vi "Func-엑셀 데이터를 그래프로 출력.vi"() -> ()   [LabVIEW 2015] (continued)
-12.31\n-18.3\t-18.31\t-12.305\n-18.3\t-18.31\t-12.3\n-18.3\t-18.31\t-12.299\n-18.3\t-18.31\t-12.293\n-18.3\t-18.31\t-12.295\n-18.3\t-18.31\t-12.293\n-18.3\t-18.31\t-12.286\n-18.3\t-18.31\t-12.284\n-18.3\t-18.31\t-12.277\n-18.3\t-18.31\t-12.27\n-18.3\t-18.31\t-12.265\n-18.3\t-18.31\t-12.259\n-18.3\t-18.31\t-12.253\n-18.3\t-18.31\t-12.251\n-18.3\t-18.31\t-12.25\n-18.3\t-18.31\t-12.245\n-18.3\t-18.31\t-12.239\n-18.3\t-18.31\t-12.232\n-18.3\t-18.31\t-12.23\n-18.3\t-18.31\t-12.226\n-18.3\t-18.31\t-12.221\n-18.3\t-18.31\t-12.22\n-18.3\t-18.31\t-12.216\n-18.3\t-18.31\t-12.214\n-18.3\t-18.31\t-12.209\n-18.3\t-18.31\t-12.205\n-18.3\t-18.31\t-12.202\n-18.3\t-18.31\t-12.199\n-18.3\t-18.31\t-12.195\n-18.3\t-18.31\t-12.192\n-18.3\t-18.31\t-12.186\n-18.3\t-18.31\t-12.184\n-18.3\t-18.31\t-12.179\n-18.3\t-18.31\t-12.169\n-18.3\t-18.31\t-12.166\n-18.3\t-18.31\t-12.161\n-18.3\t-18.31\t-12.157\n-18.3\t-18.31\t-12.152\n-18.3\t-18.31\t-12.15\n-18.3\t-18.31\t-12.146\n-18.3\t-18.31\t-12.143\n-18.3\t-18.31\t-12.142\n-18.3\t-18.31\t-12.137\n-18.3\t-18.31\t-12.132\n-18.3\t-18.31\t-12.127\n-18.3\t-18.31\t-12.123\n-18.3\t-18.31\t-12.118\n-18.3\t-18.31\t-12.112\n-18.3\t-18.31\t-12.107\n-18.3\t-18.31\t-12.105\n-18.3\t-18.31\t-12.102\n-18.3\t-18.31\t-12.097\n-18.3\t-18.31\t-12.095\n-18.3\t-18.31\t-12.093\n-18.3\t-18.31\t-12.089\n-18.3\t-18.31\t-12.083\n-18.3\t-18.31\t-12.078\n-18.3\t-18.31\t-12.071\n-18.3\t-18.31\t-12.07\n-18.3\t-18.31\t-12.066\n-18.3\t-18.31\t-12.06\n-18.3\t-18.31\t-12.057\n-18.3\t-18.31\t-12.055\n-18.3\t-18.31\t-12.053\n-18.3\t-18.31\t-12.049\n-18.3\t-18.31\t-12.049\n-18.3\t-18.31\t-12.044\n-18.3\t-18.31\t-12.04\n-18.3\t-18.31\t-12.036\n-18.3\t-18.31\t-12.028\n-18.3\t-18.31\t-12.025\n-18.3\t-18.31\t-12.021\n-18.3\t-18.31\t-12.017\n-18.3\t-18.31\t-12.013\n-18.3\t-18.31\t-12.008\n-18.3\t-18.31\t-12.003\n-18.3\t-18.31\t-11.996\n-18.3\t-18.31\t-11.993\n-18.3\t-18.31\t-11.99\n-18.3\t-18.31\t-11.989\n-18.3\t-18.31\t-11.989\n-18.3\t-18.31\t-11.988\n-18.3\t-18.31\t-11.984\n-18.3\t-18.31\t-11.975\n-18.3\t-18.31\t-11.97\n-18.3\t-18.31\t-11.965\n-18.3\t-18.31\t-11.959\n-18.3\t-18.31\t-11.952\n-18.3\t-18.31\t-11.95\n-18.3\t-18.31\t-11.947\n-18.3\t-18.31\t-11.946\n-18.3\t-18.31\t-11.943\n-18.3\t-18.31\t-11.939\n-18.3\t-18.31\t-11.937\n-18.3\t-18.31\t-11.93\n-18.3\t-18.31\t-11.925\n-18.3\t-18.31\t-11.923\n-18.3\t-18.31\t-11.921\n-18.3\t-18.31\t-11.919\n-18.3\t-18.31\t-11.914\n-18.3\t-18.31\t-11.913\n-18.3\t-18.31\t-11.905\n-18.3\t-18.31\t-11.902\n-18.3\t-18.31\t-11.896\n-18.3\t-18.31\t-11.894\n-18.3\t-18.31\t-11.892\n-18.3\t-18.31\t-11.889\n-18.3\t-18.31\t-11.891\n-18.3\t-18.31\t-11.885\n-18.3\t-18.31\t-11.88\n-18.3\t-18.31\t-11.871\n-18.3\t-18.31\t-11.868\n-18.3\t-18.31\t-11.863\n-18.3\t-18.31\t-11.86\n-18.3\t-18.31\t-11.853\n-18.3\t-18.31\t-11.85\n-18.3\t-18.31\t-11.847\n-18.3\t-18.31\t-11.842\n-18.3\t-18.31\t-11.837\n-18.3\t-18.31\t-11.831\n-18.3\t-18.31\t-11.833\n-18.3\t-18.31\t-11.829\n-18.3\t-18.31\t-11.825\n-18.3\t-18.31\t-11.824\n-18.3\t-18.31\t-11.823\n-18.3\t-18.31\t-11.82\n-18.3\t-18.31\t-11.816\n-18.3\t-18.31\t-11.816\n-18.3\t-18.31\t-11.811\n-18.3\t-18.31\t-11.806\n-18.3\t-18.31\t-11.802\n-18.3\t-18.31\t-11.797\n-18.3\t-18.31\t-11.791\n-18.3\t-18.31\t-11.786\n-18.3\t-18.31\t-11.78\n-18.3\t-18.31\t-11.777\n-18.3\t-18.31\t-11.774\n-18.3\t-18.31\t-11.77\n-18.3\t-18.31\t-11.769\n-18.3\t-18.31\t-11.766\n-18.3\t-18.31\t-11.762\n-18.3\t-18.31\t-11.759\n-18.3\t-18.31\t-11.755\n-18.3\t-18.31\t-11.751\n-18.3\t-18.31\t-11.748\n-18.3\t-18.31\t-11.742\n-18.3\t-18.31\t-11.738\n-18.3\t-18.31\t-11.736\n-18.3\t-18.31\t-11.735\n-18.3\t-18.31\t-11.729\n-18.3\t-18.31\t-11.726\n-18.3\t-18.31\t-11.727\n-18.3\t-18.31\t-11.724\n-18.3\t-18.31\t-11.72\n-18.3\t-18.31\t-11.718\n-18.3\t-18.31\t-11.715\n-18.3\t-18.31\t-11.711\n-18.3\t-18.31\t-11.701\n-18.3\t-18.31\t-11.701\n-18.3\t-18.31\t-11.697\n-18.3\t-18.31\t-11.693\n-18.3\t-18.31\t-11.686\n-18.3\t-18.31\t-11.68\n-18.3\t-18.31\t-11.68\n-18.3\t-18.31\t-11.675\n-18.3\t-18.31\t-11.671\n-18.3\t-18.31\t-11.67\n-18.3\t-18.31\t-11.668\n-18.3\t-18.31\t-11.664\n-18.3\t-18.31\t-11.66\n-18.3\t-18.31\t-11.654\n-18.3\t-18.31\t-11.652\n-18.3\t-18.31\t-11.642\n-18.3\t-18.31\t-11.641\n-18.3\t-18.31\t-11.638\n-18.3\t-18.31\t-11.634\n-18.3\t-18.31\t-11.636\n-18.3\t-18.31\t-11.634\n-18.3\t-18.31\t-11.634\n-18.3\t-18.31\t-11.63\n-18.3\t-18.31\t-11.631\n-18.3\t-18.31\t-11.624\n-18.3\t-18.31\t-11.621\n-18.3\t-18.31\t-11.618\n-18.3\t-18.31\t-11.613\n-18.3\t-18.31\t-11.607\n-18.3\t-18.31\t-11.603\n-18.3\t-18.31\t-11.6\n-18.3\t-18.31\t-11.595\n-18.3\t-18.31\t-11.595\n-18.3\t-18.31\t-11.592\n-18.3\t-18.31\t-11.591\n-18.3\t-18.31\t-11.59\n-18.3\t-18.31\t-11.587\n-18.3\t-18.31\t-11.584\n-18.3\t-18.31\t-11.579\n-18.3\t-18.31\t-11.576\n-18.3\t-18.31\t-11.569\n-18.3\t-18.31\t-11.564\n-18.3\t-18.31\t-11.561\n-18.3\t-18.31\t-11.554\n-18.3\t-18.31\t-11.55\n-18.3\t-18.31\t-11.545\n-18.3\t-18.31\t-11.543\n-18.3\t-18.31\t-11.54\n-18.3\t-18.31\t-11.536\n-18.3\t-18.31\t-11.537\n-18.3\t-18.31\t-11.536\n-18.3\t-18.31\t-11.53\n-18.3\t-18.31\t-11.527\n-18.3\t-18.31\t-11.523\n-18.3\t-18.31\t-11.518\n-18.3\t-18.31\t-11.515\n-18.3\t-18.31\t-11.511\n-18.3\t-18.31\t-11.511\n-18.3\t-18.31\t-11.506\n-18.3\t-18.31\t-11.505\n-18.3\t-18.31\t-11.502\n-18.3\t-18.31\t-11.497\n-18.3\t-18.31\t-11.495\n-18.3\t-18.31\t-11.492\n-18.3\t-18.31\t-11.489\n-18.3\t-18.31\t-11.485\n-18.3\t-18.31\t-11.483\n-18.3\t-18.31\t-11.479\n-18.3\t-18.31\t-11.472\n-18.3\t-18.31\t-11.466\n-18.3\t-18.31\t-11.463\n-18.3\t-18.31\t-11.456\n-18.3\t-18.31\t-11.451\n-18.3\t-18.31\t-11.446\n-18.3\t-18.31\t-11.444\n-18.3\t-18.31\t-11.446\n-18.3\t-18.31\t-11.44\n-18.3\t-18.31\t-11.437\n-18.3\t-18.31\t-11.437\n-18.3\t-18.31\t-11.436\n-18.3\t-18.31\t-11.432\n-18.3\t-18.31\t-11.427\n-18.3\t-18.31\t-11.422\n-18.3\t-18.31\t-11.421\n-18.3\t-18.31\t-11.418\n-18.3\t-18.31\t-11.412\n-18.3\t-18.31\t-11.409\n-18.3\t-18.31\t-11.406\n-18.3\t-18.31\t-11.404\n-18.3\t-18.31\t-11.404\n-18.3\t-18.31\t-11.401\n-18.3\t-18.31\t-11.397\n-18.3\t-18.31\t-11.396\n-18.3\t-18.31\t-11.391\n-18.3\t-18.31\t-11.383\n-18.3\t-18.31\t-11.379\n-18.3\t-18.31\t-11.38\n-18.3\t-18.31\t-11.379\n-18.3\t-18.31\t-11.376\n-18.3\t-18.31\t-11.372\n-18.3\t-18.31\t-11.375\n-18.3\t-18.31\t-11.371\n-18.3\t-18.31\t-11.364\n-18.3\t-18.31\t-11.358\n-18.3\t-18.31\t-11.352\n-18.3\t-18.31\t-11.355\n-18.3\t-18.31\t-11.35\n-18.3\t-18.31\t-11.347\n-18.3\t-18.31\t-11.345\n-18.3\t-18.31\t-11.347\n-18.3\t-18.31\t-11.346\n-18.3\t-18.31\t-11.339\n-18.3\t-18.31\t-11.336\n-18.3\t-18.31\t-11.332\n-18.3\t-18.31\t-11.327\n-18.3\t-18.31\t-11.318\n-18.3\t-18.31\t-11.316\n-18.3\t-18.31\t-11.311\n-18.3\t-18.31\t-11.305\n-18.3\t-18.31\t-11.302\n-18.3\t-18.31\t-11.302\n-18.3\t-18.31\t-11.301\n-18.3\t-18.31\t-11.299\n-18.3\t-18.31\t-11.296\n-18.3\t-18.31\t-11.292\n-18.3\t-18.31\t-11.292\n-18.3\t-18.31\t-11.289\n-18.3\t-18.31\t-11.281\n-18.3\t-18.31\t-11.276\n-18.3\t-18.31\t-11.277\n-18.3\t-18.31\t-11.279\n-18.3\t-18.31\t-11.276\n-18.3\t-18.31\t-11.271\n-18.3\t-18.31\t-11.27\n-18.3\t-18.31\t-11.269\n-18.3\t-18.31\t-11.265\n-18.3\t-18.31\t-11.258\n-18.3\t-18.31\t-11.254\n-18.3\t-18.31\t-11.255\n-18.3\t-18.31\t-11.252\n-18.3\t-18.31\t-11.25\n-18.3\t-18.31\t-11.249\n-18.3\t-18.31\t-11.242\n-18.3\t-18.31\t-11.237\n-18.3\t-18.31\t-11.233\n-18.3\t-18.31\t-11.23\n-18.3\t-18.31\t-11.227\n-18.3\t-18.31\t-11.222\n-18.3\t-18.31\t-11.222\n-18.3\t-18.31\t-11.221\n-18.3\t-18.31\t-11.218\n-18.3\t-18.31\t-11.214\n-18.3\t-18.31\t-11.212\n-18.3\t-18.31\t-11.21\n-18.3\t-18.31\t-11.204\n-18.3\t-18.31\t-11.2\n-18.3\t-18.31\t-11.198\n-18.3\t-18.31\t-11.194\n-18.3\t-18.31\t-11.191\n-18.3\t-18.31\t-11.187\n-18.3\t-18.31\t-11.184\n-18.3\t-18.31\t-11.188\n-18.3\t-18.31\t-11.183\n-18.3\t-18.31\t-11.179\n-18.3\t-18.31\t-11.175\n-18.3\t-18.31\t-11.17\n-18.3\t-18.31\t-11.166\n-18.3\t-18.31\t-11.156\n-18.3\t-18.31\t-11.151\n-18.3\t-18.31\t-11.147\n-18.3\t-18.31\t-11.146\n-18.3\t-18.31\t-11.144\n-18.3\t-18.31\t-11.141\n-18.3\t-18.31\t-11.141\n-18.3\t-18.31\t-11.137\n-18.3\t-18.31\t-11.134\n-18.3\t-18.31\t-11.128\n-18.3\t-18.31\t-11.121\n-18.3\t-18.31\t-11.121\n-18.3\t-18.31\t-11.118\n-18.3\t-18.31\t-11.118\n-18.3\t-18.31\t-11.115\n-18.3\t-18.31\t-11.114\n-18.3\t-18.31\t-11.11\n-18.3\t-18.31\t-11.106\n-18.3\t-18.31\t-11.102\n-18.3\t-18.31\t-11.094\n-18.3\t-18.31\t-11.093\n-18.3\t-18.31\t-11.091\n-18.3\t-18.31\t-11.089\n-18.3\t-18.31\t-11.085\n-18.3\t-18.31\t-11.083\n-18.3\t-18.31\t-11.079\n-18.3\t-18.31\t-11.075\n-18.3\t-18.31\t-11.071\n-18.3\t-18.31\t-11.073\n-18.3\t-18.31\t-11.067\n-18.3\t-18.31\t-11.066\n-18.3\t-18.31\t-11.064\n-18.3\t-18.31\t-11.059\n-18.3\t-18.31\t-11.056\n-18.3\t-18.31\t-11.049\n-18.3\t-18.31\t-11.048\n-18.3\t-18.31\t-11.043\n-18.3\t-18.31\t-11.037\n-18.3\t-18.31\t-11.033\n-18.3\t-18.31\t-11.029\n-18.3\t-18.31\t-11.027\n-18.3\t-18.31\t-11.026\n-18.3\t-18.31\t-11.022\n-18.3\t-18.31\t-11.025\n-18.3\t-18.31\t-11.025\n-18.3\t-18.31\t-11.024\n-18.3\t-18.31\t-11.02\n-18.3\t-18.31\t-11.016\n-18.3\t-18.31\t-11.012\n-18.3\t-18.31\t-11.007\n-18.3\t-18.31\t-11.006\n-18.3\t-18.31\t-11.001\n-18.3\t-18.31\t-10.998\n-18.3\t-18.31\t-10.994\n-18.3\t-18.31\t-10.989\n-18.3\t-18.31\t-10.984\n-18.3\t-18.31\t-10.978\n-18.3\t-18.31\t-10.974\n-18.3\t-18.31\t-10.974\n-18.3\t-18.31\t-10.975\n-18.3\t-18.31\t-10.969\n-18.3\t-18.31\t-10.967\n-18.3\t-18.31\t-10.967\n-18.3\t-18.31\t-10.959\n-18.3\t-18.31\t-10.954\n-18.3\t-18.31\t-10.95\n-18.3\t-18.31\t-10.948\n-18.3\t-18.31\t-10.945\n-18.3\t-18.31\t-10.943\n-18.3\t-18.31\t-10.941\n-18.3\t-18.31\t-10.937\n-18.3\t-18.31\t-10.934\n-18.3\t-18.31\t-10.93\n-18.3\t-18.31\t-10.928\n-18.3\t-18.31\t-10.921\n-18.3\t-18.31\t-10.919\n-18.3\t-18.31\t-10.918\n-18.3\t-18.31\t-10.914\n-18.3\t-18.31\t-10.914\n-18.3\t-18.31\t-10.914\n-18.3\t-18.31\t-10.913\n-18.3\t-18.31\t-10.908\n-18.3\t-18.31\t-10.902\n-18.3\t-18.31\t-10.899\n-18.3\t-18.31\t-10.892\n-18.3\t-18.31\t-10.888\n-18.3\t-18.31\t-10.886\n-18.3\t-18.31\t-10.886\n-18.3\t-18.31\t-10.885\n-18.3\t-18.31\t-10.881\n-18.3\t-18.31\t-10.877\n-18.3\t-18.31\t-10.877\n-18.3\t-18.31\t-10.872\n-18.3\t-18.31\t-10.868\n-18.3\t-18.31\t-10.869\n-18.3\t-18.31\t-10.867\n-18.3\t-18.31\t-10.866\n-18.3\t-18.31\t-10.861\n-18.3\t-18.31\t-10.862\n-18.3\t-18.31\t-10.857\n-18.3\t-18.31\t-10.854\n-18.3\t-18.31\t-10.851\n-18.3\t-18.31\t-10.849\n-18.3\t-18.31\t-10.848\n-18.3\t-18.31\t-10.843\n-18.3\t-18.31\t-10.84\n-18.3\t-18.31\t-10.837\n-18.3\t-18.31\t-10.835\n-18.3\t-18.31\t-10.829\n-18.3\t-18.31\t-10.824\n-18.3\t-18.31\t-10.824\n-18.3\t-18.31\t-10.819\n-18.3\t-18.31\t-10.812\n-18.3\t-18.31\t-10.811\n-18.3\t-18.31\t-10.809\n-18.3\t-18.31\t-10.804\n-18.3\t-18.31\t-10.797\n-18.3\t-18.31\t-10.797\n-18.3\t-18.31\t-10.797\n-18.3\t-18.31\t-10.795\n-18.3\t-18.31\t-10.793\n-18.3\t-18.31\t-10.794\n-18.3\t-18.31\t-10.796\n-18.3\t-18.31\t-10.795\n-18.3\t-18.31\t-10.792\n-18.3\t-18.31\t-10.786\n-18.3\t-18.31\t-10.783\n-18.3\t-18.31\t-10.779\n-18.3\t-18.31\t-10.77\n-18.3\t-18.31\t-10.766\n-18.3\t-18.31\t-10.762\n-18.3\t-18.31\t-10.762\n-18.3\t-18.31\t-10.76\n-18.3\t-18.31\t-10.756\n-18.3\t-18.31\t-10.755\n-18.3\t-18.31\t-10.753\n-18.3\t-18.31\t-10.752\n-18.3\t-18.31\t-10.745\n-18.3\t-18.31\t-10.743\n-18.3\t-18.31\t-10.743\n-18.3\t-18.31\t-10.738\n-18.3\t-18.31\t-10.738\n-18.3\t-18.31\t-10.737\n-18.3\t-18.31\t-10.738\n-18.3\t-18.31\t-10.734\n-18.3\t-18.31\t-10.73\n-18.3\t-18.31\t-10.728\n-18.3\t-18.31\t-10.725\n-18.3\t-18.31\t-10.72\n-18.3\t-18.31\t-10.717\n-18.3\t-18.31\t-10.714\n-18.3\t-18.31\t-10.707\n-18.3\t-18.31\t-10.705\n-18.3\t-18.31\t-10.704\n-18.3\t-18.31\t-10.702\n-18.3\t-18.31\t-10.698\n-18.3\t-18.31\t-10.698\n-18.3\t-18.31\t-10.696\n-18.3\t-18.31\t-10.697\n-18.3\t-18.31\t-10.687\n-18.3\t-18.31\t-10.683\n-18.3\t-18.31\t-10.68\n-18.3\t-18.31\t-10.678\n-18.3\t-18.31\t-10.676\n-18.3\t-18.31\t-10.673\n-18.3\t-18.31\t-10.676\n-18.3\t-18.31\t-10.673\n-18.3\t-18.31\t-10.671\n-18.3\t-18.31\t-10.664\n-18.3\t-18.31\t-10.662\n-18.3\t-18.31\t-10.658\n-18.3\t-18.31\t-10.655\n-18.3\t-18.31\t-10.654\n-18.3\t-18.31\t-10.65\n-18.3\t-18.31\t-10.65\n-18.3\t-18.31\t-10.645\n-18.3\t-18.31\t-10.646\n-18.3\t-18.31\t-10.643\n-18.3\t-18.31\t-10.636\n-18.3\t-18.31\t-10.64\n-18.3\t-18.31\t-10.641\n-18.3\t-18.31\t-10.635\n-18.3\t-18.31\t-10.631\n-18.3\t-18.31\t-10.63\n-18.3\t-18.31\t-10.629\n-18.3\t-18.31\t-10.624\n-18.3\t-18.31\t-10.621\n-18.3\t-18.31\t-10.62\n-18.3\t-18.31\t-10.618\n-18.3\t-18.31\t-10.615\n-18.3\t-18.31\t-10.615\n-18.3\t-18.31\t-10.613\n-18.3\t-18.31\t-10.608\n-18.3\t-18.31\t-10.607\n-18.3\t-18.31\t-10.607\n-18.3\t-18.31\t-10.605\n-18.3\t-18.31\t-10.602\n-18.3\t-18.31\t-10.598\n-18.3\t-18.31\t-10.599\n-18.3\t-18.31\t-10.595\n-18.3\t-18.31\t-10.591\n-18.3\t-18.31\t-10.588\n-18.3\t-18.31\t-10.586\n-18.3\t-18.31\t-10.585\n-18.3\t-18.31\t-10.581\n-18.3\t-18.31\t-10.576\n-18.3\t-18.31\t-10.574\n-18.3\t-18.31\t-10.572\n-18.3\t-18.31\t-10.569\n-18.3\t-18.31\t-10.567\n-18.3\t-18.31\t-10.564\n-18.3\t-18.31\t-10.562\n-18.3\t-18.31\t-10.562\n-18.3\t-18.31\t-10.559\n-18.3\t-18.31\t-10.557\n-18.3\t-18.31\t-10.553\n-18.3\t-18.31\t-10.552\n-18.3\t-18.31\t-10.552\n-18.3\t-18.31\t-10.55\n-18.3\t-18.31\t-10.549\n-18.3\t-18.31\t-10.545\n-18.3\t-18.31\t-10.542\n-18.3\t-18.31\t-10.542\n-18.3\t-18.31\t-10.534\n-18.3\t-18.31\t-10.529\n-18.3\t-18.31\t-10.526\n-18.3\t-18.31\t-10.523\n-18.3\t-18.31\t-10.523\n-18.3\t-18.31\t-10.519\n-18.3\t-18.31\t-10.519\n-18.3\t-18.31\t-10.519\n-18.3\t-18.31\t-10.52\n-18.3\t-18.31\t-10.517\n-18.3\t-18.31\t-10.515\n-18.3\t-18.31\t-10.513\n-18.3\t-18.31\t-10.512\n-18.3\t-18.31\t-10.505\n-18.3\t-18.31\t-10.498\n-18.3\t-18.31\t-10.494\n-18.3\t-18.31\t-10.495\n-18.3\t-18.31\t-10.496\n-18.3\t-18.31\t-10.494\n-18.3\t-18.31\t-10.496\n-18.3\t-18.31\t-10.498\n-18.3\t-18.31\t-10.499\n-18.3\t-18.31\t-10.494\n-18.3\t-18.31\t-10.488\n-18.3\t-18.31\t-10.484\n-18.3\t-18.31\t-10.481\n-18.3\t-18.31\t-10.476\n-18.3\t-18.31\t-10.471\n-18.3\t-18.31\t-10.47\n-18.3\t-18.31\t-10.471\n-18.3\t-18.31\t-10.471\n-18.3\t-18.31\t-10.468\n-18.3\t-18.31\t-10.468\n-18.3\t-18.31\t-10.464\n-18.3\t-18.31\t-10.461\n-18.3\t-18.31\t-10.461\n-18.3\t-18.31\t-10.453\n-18.3\t-18.31\t-10.454\n-18.3\t-18.31\t-10.45\n-18.3\t-18.31\t-10.45\n-18.3\t-18.31\t-10.45\n-18.3\t-18.31\t-10.445\n-18.3\t-18.31\t-10.446\n-18.3\t-18.31\t-10.44\n-18.3\t-18.31\t-10.438\n-18.3\t-18.31\t-10.438\n-18.3\t-18.31\t-10.431\n-18.3\t-18.31\t-10.429\n-18.3\t-18.31\t-10.425\n-18.3\t-18.31\t-10.428\n-18.3\t-18.31\t-10.427\n-18.3\t-18.31\t-10.424\n-18.3\t-18.31\t-10.425\n-18.3\t-18.31\t-10.425\n-18.3\t-18.31\t-10.424\n-18.3\t-18.31\t-10.421\n-18.3\t-18.31\t-10.42\n-18.3\t-18.31\t-10.416\n-18.3\t-18.31\t-10.418\n-18.3\t-18.31\t-10.414\n-18.3\t-18.31\t-10.412\n-18.3\t-18.31\t-10.41\n-18.3\t-18.31\t-10.411\n-18.3\t-18.31\t-10.405\n-18.3\t-18.31\t-10.404\n-18.3\t-18.31\t-10.403\n-18.3\t-18.31\t-10.399\n-18.3\t-18.31\t-10.398\n-18.3\t-18.31\t-10.396\n-18.3\t-18.31\t-10.393\n-18.3\t-18.31\t-10.39\n-18.3\t-18.31\t-10.39\n-18.3\t-18.31\t-10.388\n-18.3\t-18.31\t-10.387\n-18.3\t-18.31\t-10.383\n-18.3\t-18.31\t-10.382\n-18.3\t-18.31\t-10.379\n-18.3\t-18.31\t-10.374\n-18.3\t-18.31\t-10.369\n-18.3\t-18.31\t-10.366\n-18.3\t-18.31\t-10.362\n-18.3\t-18.31\t-10.36\n-18.3\t-18.31\t-10.36\n-18.3\t-18.31\t-10.359\n-18.3\t-18.31\t-10.358\n-18.3\t-18.31\t-10.352\n-18.3\t-18.31\t-10.351\n-18.3\t-18.31\t-10.35\n-18.3\t-18.31\t-10.344\n-18.3\t-18.31\t-10.342\n-18.3\t-18.31\t-10.342\n-18.3\t-18.31\t-10.344\n-18.3\t-18.31\t-10.343\n-18.3\t-18.31\t-10.339\n-18.3\t-18.31\t-10.339\n-18.3\t-18.31\t-10.339\n-18.3\t-18.31\t-10.336\n-18.3\t-18.31\t-10.335\n-18.3\t-18.31\t-10.335\n-18.3\t-18.31\t-10.333\n-18.3\t-18.31\t-10.334\n-18.3\t-18.31\t-10.329\n-18.3\t-18.31\t-10.329\n-18.3\t-18.31\t-10.325\n-18.3\t-18.31\t-10.322\n-18.3\t-18.31\t-10.321\n-18.3\t-18.31\t-10.317\n-18.3\t-18.31\t-10.315\n-18.3\t-18.31\t-10.312\n-18.3\t-18.31\t-10.31\n-18.3\t-18.31\t-10.308\n-18.3\t-18.31\t-10.306\n-18.3\t-18.31\t-10.304\n-18.3\t-18.31\t-10.301\n-18.3\t-18.31\t-10.298\n-18.3\t-18.31\t-10.298\n-18.3\t-18.31\t-10.295\n-18.3\t-18.31\t-10.292\n-18.3\t-18.31\t-10.291\n-18.3\t-18.31\t-10.292\n-18.3\t-18.31\t-10.289\n-18.3\t-18.31\t-10.286\n-18.3\t-18.31\t-10.286\n-18.3\t-18.31\t-10.282\n-18.3\t-18.31\t-10.279\n-18.3\t-18.31\t-10.275\n-18.3\t-18.31\t-10.27\n-18.3\t-18.31\t-10.271\n-18.3\t-18.31\t-10.271\n-18.3\t-18.31\t-10.268\n-18.3\t-18.31\t-10.27\n-18.3\t-18.31\t-10.269\n-18.3\t-18.31\t-10.273\n-18.3\t-18.31\t-10.269\n-18.3\t-18.31\t-10.266\n-18.3\t-18.31\t-10.265\n-18.3\t-18.31\t-10.263\n-18.3\t-18.31\t-10.262\n-18.3\t-18.31\t-10.255\n-18.3\t-18.31\t-10.252\n-18.3\t-18.31\t-10.25\n-18.3\t-18.31\t-10.246\n-18.3\t-18.31\t-10.244\n-18.3\t-18.31\t-10.242\n-18.3\t-18.31\t-10.241\n-18.3\t-18.31\t-10.245\n-18.3\t-18.31\t-10.243\n-18.3\t-18.31\t-10.245\n-18.3\t-18.31\t-10.243\n-18.3\t-18.31\t-10.239\n-18.3\t-18.31\t-10.239\n-18.3\t-18.31\t-10.235\n-18.3\t-18.31\t-10.233\n-18.3\t-18.31\t-10.229\n-18.3\t-18.31\t-10.225\n-18.3\t-18.31\t-10.227\n-18.3\t-18.31\t-10.222\n-18.3\t-18.31\t-10.221\n-18.3\t-18.31\t-10.218\n-18.3\t-18.31\t-10.215\n-18.3\t-18.31\t-10.216\n-18.3\t-18.31\t-10.214\n-18.3\t-18.31\t-10.213\n-18.3\t-18.31\t-10.211\n-18.3\t-18.31\t-10.212\n-18.3\t-18.31\t-10.209\n-18.3\t-18.31\t-10.207\n-18.3\t-18.31\t-10.204\n-18.3\t-18.31\t-10.199\n-18.3\t-18.31\t-10.196\n-18.3\t-18.31\t-10.198\n-18.3\t-18.31\t-10.198\n-18.3\t-18.31\t-10.199\n-18.3\t-18.31\t-10.199\n-18.3\t-18.31\t-10.197\n-18.3\t-18.31\t-10.196\n-18.3\t-18.31\t-10.19\n-18.3\t-18.31\t-10.189\n-18.3\t-18.31\t-10.187\n-18.3\t-18.31\t-10.186\n-18.3\t-18.31\t-10.185\n-18.3\t-18.31\t-10.182\n-18.3\t-18.31\t-10.182\n-18.3\t-18.31\t-10.18\n-18.3\t-18.31\t-10.177\n-18.3\t-18.31\t-10.177\n-18.3\t-18.31\t-10.176\n-18.3\t-18.31\t-10.175\n-18.3\t-18.31\t-10.179\n-18.3\t-18.31\t-10.173\n-18.3\t-18.31\t-10.172\n-18.3\t-18.31\t-10.166\n-18.3\t-18.31\t-10.165\n-18.3\t-18.31\t-10.163\n-18.3\t-18.31\t-10.159\n-18.3\t-18.31\t-10.155\n-18.3\t-18.31\t-10.152\n-18.3\t-18.31\t-10.15\n-18.3\t-18.31\t-10.15\n-18.3\t-18.31\t-10.148\n-18.3\t-18.31\t-10.151\n-18.3\t-18.31\t-10.151\n-18.3\t-18.31\t-10.152\n-18.3\t-18.31\t-10.15\n-18.3\t-18.31\t-10.146\n-18.3\t-18.31\t-10.146\n-18.3\t-18.31\t-10.14\n-18.3\t-18.31\t-10.139\n-18.3\t-18.31\t-10.137\n-18.3\t-18.31\t-10.137\n-18.3\t-18.31\t-10.136\n-18.3\t-18.31\t-10.132\n-18.3\t-18.31\t-10.128\n-18.3\t-18.31\t-10.123\n-18.3\t-18.31\t-10.12\n-18.3\t-18.31\t-10.119\n-18.3\t-18.31\t-10.118\n-18.3\t-18.31\t-10.118\n-18.3\t-18.31\t-10.117\n-18.3\t-18.31\t-10.119\n-18.3\t-18.31\t-10.116\n-18.3\t-18.31\t-10.113\n-18.3\t-18.31\t-10.112\n-18.3\t-18.31\t-10.109\n-18.3\t-18.31\t-10.108\n-18.3\t-18.31\t-10.109\n-18.3\t-18.31\t-10.109\n-18.3\t-18.31\t-10.105\n-18.3\t-18.31\t-10.104\n-18.3\t-18.31\t-10.103\n-18.3\t-18.31\t-10.101\n-18.3\t-18.31\t-10.097\n-18.3\t-18.31\t-10.093\n-18.3\t-18.31\t-10.093\n-18.3\t-18.31\t-10.092\n-18.3\t-18.31\t-10.093\n-18.3\t-18.31\t-10.091\n-18.3\t-18.31\t-10.089\n-18.3\t-18.31\t-10.092\n-18.3\t-18.31\t-10.091\n-18.3\t-18.31\t-10.086\n-18.3\t-18.31\t-10.083\n-18.3\t-18.31\t-10.08\n-18.3\t-18.31\t-10.078\n-18.3\t-18.31\t-10.074\n-18.3\t-18.31\t-10.072\n-18.3\t-18.31\t-10.072\n-18.3\t-18.31\t-10.073\n-18.3\t-18.31\t-10.075\n-18.3\t-18.31\t-10.073\n-18.3\t-18.31\t-10.071\n-18.3\t-18.31\t-10.069\n-18.3\t-18.31\t-10.07\n-18.3\t-18.31\t-10.07\n-18.3\t-18.31\t-10.061\n-18.3\t-18.31\t-10.061\n-18.3\t-18.31\t-10.059\n-18.3\t-18.31\t-10.059\n-18.3\t-18.31\t-10.056\n-18.3\t-18.31\t-10.054\n-18.3\t-18.31\t-10.056\n-18.3\t-18.31\t-10.054\n-18.3\t-18.31\t-10.055\n-18.3\t-18.31\t-10.048\n-18.3\t-18.31\t-10.049\n-18.3\t-18.31\t-10.05\n-18.3\t-18.31\t-10.047\n-18.3\t-18.31\t-10.046\n-18.3\t-18.31\t-10.046\n-18.3\t-18.31\t-10.05\n-18.3\t-18.31\t-10.05\n-18.3\t-18.31\t-10.045\n-18.3\t-18.31\t-10.042\n-18.3\t-18.31\t-10.042\n-18.3\t-18.31\t-10.041\n-18.3\t-18.31\t-10.039\n-18.3\t-18.31\t-10.034\n-18.3\t-18.31\t-10.032\n-18.3\t-18.31\t-10.031\n-18.3\t-18.31\t-10.03\n-18.3\t-18.31\t-10.027\n-18.3\t-18.31\t-10.022\n-18.3\t-18.31\t-10.022\n-18.3\t-18.31\t-10.023\n-18.3\t-18.31\t-10.023\n-18.3\t-18.31\t-10.022\n-18.3\t-18.31\t-10.021\n-18.3\t-18.31\t-10.017\n-18.3\t-18.31\t-10.016\n-18.3\t-18.31\t
